vi "DSF.Engine.Transfer.Set String Buffer.vi"(10 "Buffer":refnum<class "Memory Buffer.lvclass">, 11 "Transfer in":refnum<class "DSF.Engine.Transfer.lvclass">) -> (3 "Transfer out":refnum<class "DSF.Engine.Transfer.lvclass">)   [LabVIEW 2017, in "Data Sharing Framework Engine.lvlib" / "DSF.Engine.Transfer.lvclass"]
uses:
  DSF.Engine.Transfer.lvclass
  Source/Data Sharing Framework Core/Engine/Memory/Memory Buffer/Memory Buffer.lvclass
  DSF.Engine.Transfer.lvclass/DSF.Engine.Transfer.ctl
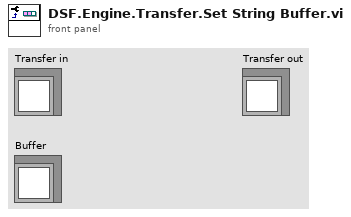
[diagram p1: front panel]
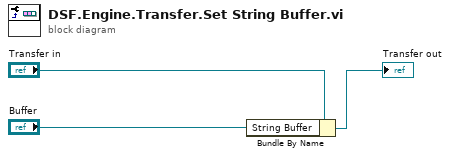
[diagram p0: block diagram]
diagram:
  n1 = Bundle By Name(cluster="Transfer in", "String Buffer"="Buffer") -> (→"Transfer out":refnum<class "DSF.Engine.Transfer.lvclass">)
